vi "VCI_ERR_INFO_1_CONVERT.vi"(1 "VCI_ERR_INFO_1":T2) -> (0 "VCI_ERR_INFO":T1)   [LabVIEW 2018, in "ControlCan.lvlib"]
uses:
  ControlCan.lvlib
  VCI_ERR_INFO_1.ctl
  VCI_ERR_INFO.ctl
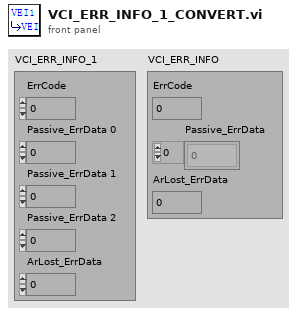
[diagram p1: front panel]
types:
  T1 = typedef "ControlCAN.lvlib/VCI_ERR_INFO.ctl" = cluster{"ErrCode":u32, "Passive_ErrData":u8[], "ArLost_ErrData":u8}
  T2 = typedef "ControlCAN.lvlib/VCI_ERR_INFO_1.ctl" = cluster{"ErrCode":u32, "Passive_ErrData 0":u8, "Passive_ErrData 1":u8, "Passive_ErrData 2":u8, "ArLost_ErrData":u8}
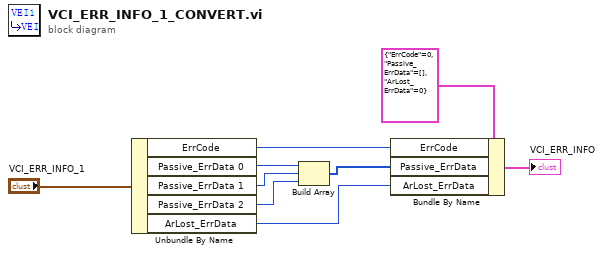
[diagram p0: block diagram]
diagram:
  n1 = Unbundle By Name("VCI_ERR_INFO_1") -> ("ErrCode"=w7:u32, "Passive_ErrData 0"=w6:u8, "Passive_ErrData 1"=w5:u8, "Passive_ErrData 2"=w4:u8, "ArLost_ErrData"=w2:u8)
  n2 = Build Array(w6, w5, w4) -> (w3:u8[])
  n3 = Bundle By Name(cluster=T1 {"ErrCode"=0, "Passive_ErrData"=[], "ArLost_ErrData"=0} ("VCI_ERR_INFO"), "ErrCode"=w7, "Passive_ErrData"=w3, "ArLost_ErrData"=w2) -> (→"VCI_ERR_INFO":T1)
